vi "Global_HW Data.vi"() -> ()   [LabVIEW 2017, in "Joystick.lvlib"]
uses:
  Joystick/Joystick.lvlib
panel:
  in  "JoystickHW_USB1 Buttons":bool[](array[boolean])
  in  "JoystickHW_USB1 Axes":dbl[](array[numeric])
  in  "JoystickHW_USB0 Buttons":bool[](array[boolean])
  in  "JoystickHW_USB0 Axes":dbl[](array[numeric])
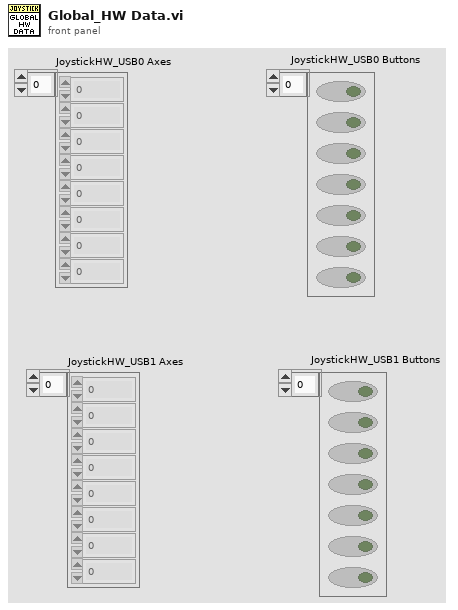
[diagram p1: front panel]
diagram:
